vi "p1.vi"() -> ()   [LabVIEW 2023, in "d19.lvlib"]
uses:
  d19.lvlib
  Users/Standard/OneDrive - Argenta/Desktop/SubPanel Actors/GUI/GUI/Rule Type.ctl
  <vilib>/regexp/Match Regular Expression.xnode
  AOC/AOC.lvlib
panel:
  in  "Example":string="px{a<2006:qkq,m>2090:A,rfg}\npv{a>1716:R,A}\nlnx{m>1548:A,A}\nrfg{s<537:gd,x>2440:R,A}\nqs{s>3448:A,lnx}\nqkq{x<1416:A,crn}\ncrn{x>2662:A,R}\nin{s<1351:px,qqz}\nqqz{s>2770:qs,m<1801:hdj,R}\ngd{a>3333:R,R}\nhdj{m>838:A,pv}\n\n{x=787,m=2655,a=1222,s=2876}\n{x=1679,m=44,a=2067,s=496}\n{x=2036,m=264,a=79,s=2244}\n{x=2461,m=1339,a=466,s=291}\n{x=2127,m=1623,a=2188,s=1013}"
  in  "Example":bool=TRUE
  out "Answer":i64=978
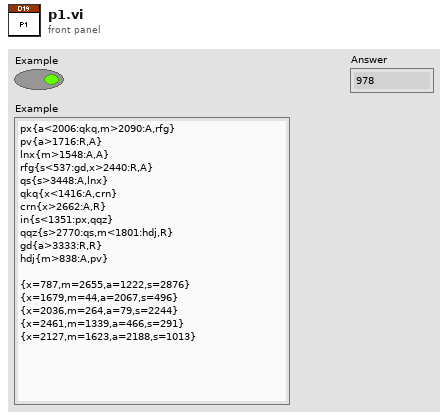
[diagram p1: front panel]
types:
  T1 = cluster{"Rule Type":string, "Index":i32, "Label":string}[]
  T2 = typedef "d19.lvlib/Rule Type.ctl" = enum16{"<", ">", "R", "A", "goto"}
  T3 = map{string, cluster{"Type":T2, "Route":string, "Rating":u8, "Value":i32}[]}
  T4 = cluster{"Type":T2, "whole match":string, "default value 1":u8, i32}
  T5 = cluster{"Type":T2, "Route":string, "Rating":u8, "Value":i32}[]
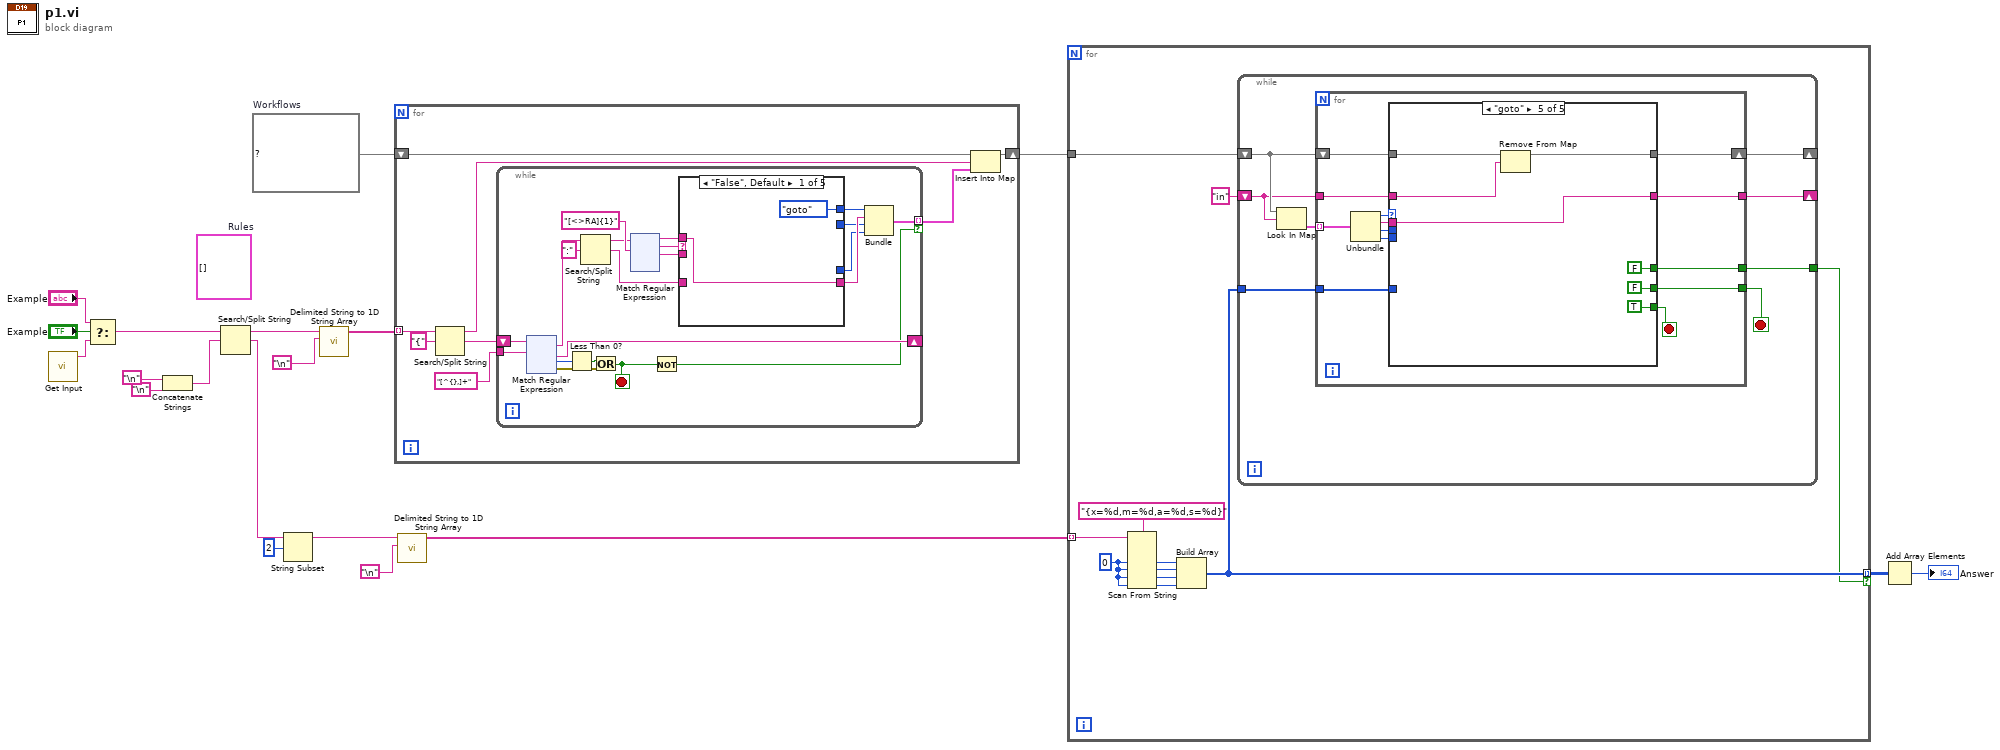
[diagram p0: block diagram]
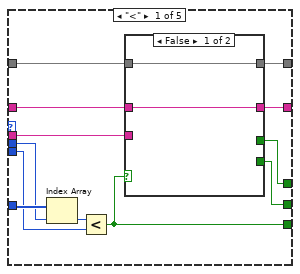
[diagram p2: hidden frame]
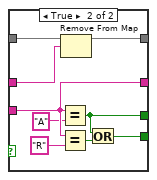
[diagram p3: hidden frame]
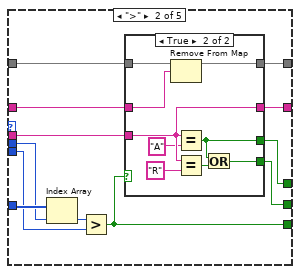
[diagram p4: hidden frame]
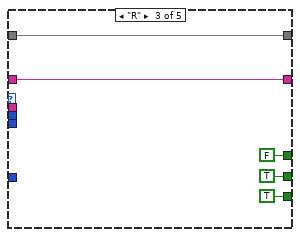
[diagram p6: hidden frame]
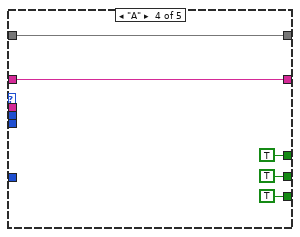
[diagram p7: hidden frame]
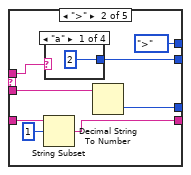
[diagram p8: hidden frame]
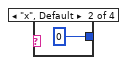
[diagram p9: hidden frame]
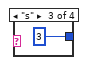
[diagram p10: hidden frame]
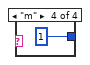
[diagram p11: hidden frame]
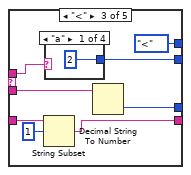
[diagram p12: hidden frame]
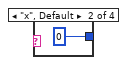
[diagram p13: hidden frame]
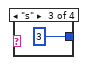
[diagram p14: hidden frame]
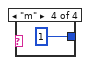
[diagram p15: hidden frame]
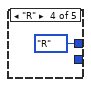
[diagram p16: hidden frame]
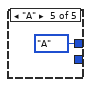
[diagram p17: hidden frame]
diagram:
  (unwired) T1 []  # Rules
  w9 = T3 {}  # Workflows
  n1 = call "Get Input.vi"() -> ("Input"=w19:string)  [unwired: 11 in]
  n2 = Select(t="Example", s="Example", f=w19) -> (s? t:f=w16:string)
  n3 = Concatenate Strings("\n", "\n") -> (w13:string)
  n4 = Search/Split String(string=w16, search string/char (-)=w13) -> (substring before match=w12:string, match + rest of string=w11:string)  [unwired: 1 in, 1 out]
  n5 = String Subset(string=w11, offset (0)=2) -> (substring=w2:string)  [unwired: 1 in]
  n6 = call <vilib>:"Delimited String to 1D String Array.vi"("delimiter"="\n", "delimited string"=w12) -> ("string array"=w10:string[])  [unwired: 9 in]
  n7 = for {
    tunnel: w10 -> [w25] mode=indexing
    shift-right: [w26] -> w5
    shift-left: w9 -> [w27]
    n8 = Search/Split String(string=w25, search string/char (-)="{") -> (substring before match=w23:string, match + rest of string=w22:string)  [unwired: 1 in, 1 out]
    n9 = while {
      shift-right: [w47] -> _
      shift-left: w22 -> [w48]
      tunnel: [w32] -> w20 mode=indexing if=w41
      tunnel: "[^{},]+" -> [w46]
      stop <- w42 stop-if-true
      n10 = xnode "Match Regular Expression"("input string"=w48, "regular expression"=w46) -> ("whole match"=w30:string, "after match"=w47:string, "offset past match"=w45:i32, "error out"=w43:errorcluster)  [unwired: 4 in, 1 out]
      n11 = Less Than 0?(x=w45) -> (x < 0?=w44:bool)
      n12 = Search/Split String(string=w30, search string/char (-)=":") -> (substring before match=w29:string, match + rest of string=w28:string)  [unwired: 1 in, 1 out]
      n13 = Or(x=w44, y=w43) -> (x .or. y?=w42:bool)
      n14 = xnode "Match Regular Expression"("input string"=w29, "regular expression"="[<>RA]{1}") -> ("before match"=w38:string, "whole match"=w39:string, "after match"=w37:string)  [unwired: 4 in, 2 out]
      n15 = Not(x=w42) -> (.not. x?=w41:bool)
      n16 = case shown="\"False\", Default" w39 {
        tunnel: [Rule_Type."goto" ("Type") Rule_Type.">" ("Type") Rule_Type."<" ("Type") Rule_Type."R" ("Type") Rule_Type."A" ("Type")] -> w36
        tunnel: w38 -> [w50 w56 w68 _ _]
        tunnel: w37 -> [_ w54 w66 _ _]
        tunnel: [_ w55 w67 _ _] -> w34
        tunnel: [_ w57 w69 _ _] -> w33
        tunnel: [w50 w52 w64 _ _] -> w35
        tunnel: w28 -> [_ w53 w65 _ _]
        frame "False", Default {
        }
        frame ">" {
          n17 = String Subset(string=w53, offset (0)=1) -> (substring=w52:string)  [unwired: 1 in]
          n18 = case shown="\"a\"" w56 {
            tunnel: [u8 2 ("default value 1") u8 0 ("default value 1") u8 3 ("default value 1") u8 1 ("default value 1")] -> w55
            frame "a" {
            }
            frame "x", Default {
            }
            frame "s" {
            }
            frame "m" {
            }
          }
          n19 = Decimal String To Number(string=w54) -> (number=w57:i32)  [unwired: 2 in, 1 out]
        }
        frame "<" {
          n20 = String Subset(string=w65, offset (0)=1) -> (substring=w64:string)  [unwired: 1 in]
          n21 = case shown="\"a\"" w68 {
            tunnel: [u8 2 ("default value 1") u8 0 ("default value 1") u8 3 ("default value 1") u8 1 ("default value 1")] -> w67
            frame "a" {
            }
            frame "x", Default {
            }
            frame "s" {
            }
            frame "m" {
            }
          }
          n22 = Decimal String To Number(string=w66) -> (number=w69:i32)  [unwired: 2 in, 1 out]
        }
        frame "R" {
        }
        frame "A" {
        }
      }
      n23 = Bundle("Type"=w36, "whole match"=w35, "default value 1"=w34, w33) -> (w32:T4)  [unwired: 1 in]
    }
    n24 = Insert Into Map(map in=w27, key=w23, value=w20) -> (map out=w26:T3)  [unwired: 2 out]
  }
  n25 = call <vilib>:"Delimited String to 1D String Array.vi"("delimiter"="\n", "delimited string"=w2) -> ("string array"=w8:string[])  [unwired: 9 in]
  n26 = for {
    tunnel: w8 -> [w321] mode=indexing
    tunnel: w5 -> [w319]
    tunnel: [w312] -> w4 mode=indexing if=w311
    w313 = i64 0 ("default value 1")
    n27 = Scan From String(format string="{x=%d,m=%d,a=%d,s=%d}", input string=w321, default 1=w313, default 2=w313, default 3=w313, default 4=w313) -> (output 1=w317:i64, output 2=w316:i64, output 3=w315:i64, output 4=w314:i64)  [unwired: 2 in, 3 out]
    n28 = Build Array(w317, w316, w315, w314) -> (w312:i64[])
    n29 = while {
      shift-right: [w327] -> _
      shift-left: "in" -> [w326]
      shift-right: [w322] -> _
      shift-left: w319 -> [w328]
      tunnel: w312 -> [w325]
      tunnel: [w323] -> w311
      stop <- w324 stop-if-true
      n30 = Look In Map(map=w328, key=w326) -> (value=w329:T5)  [unwired: 1 in, 1 out]
      n31 = for {
        tunnel: w329 -> [w342] mode=indexing
        tunnel: w325 -> [w333]
        shift-right: [w330] -> w322
        shift-left: w328 -> [w337]
        tunnel: [w336] -> w327
        tunnel: w326 -> [w334]
        tunnel: [w332] -> w324
        tunnel: [w331] -> w323
        stop <- w335 stop-if-true
        n32 = Unbundle(w342) -> ("Type"=w341:T2, "Route"=w340:string, "Rating"=w339:u8, "Value"=w338:i32)
        n33 = case shown="\"goto\"" w341 {
          tunnel: w333 -> [w354 w377 _ _ _]
          tunnel: w340 -> [w350 w373 _ _ w402]
          tunnel: w339 -> [w353 w376 _ _ _]
          tunnel: w338 -> [w351 w374 _ _ _]
          tunnel: w337 -> [w344 w367 w389 w394 w401]
          tunnel: [w349 w372 w390 w395 w402] -> w336
          tunnel: [w348 w371 TRUE TRUE TRUE] -> w335
          tunnel: w334 -> [w347 w370 w390 w395 w399]
          tunnel: [w345 w368 TRUE TRUE FALSE] -> w332
          tunnel: [w346 w369 FALSE TRUE FALSE] -> w331
          tunnel: [w343 w366 w389 w394 w400] -> w330
          frame "<" {
            n34 = Index Array(array=w354, index=w353) -> (element=w352:i64)
            n35 = Less?(x=w352, y=w351) -> (x < y?=w348:bool)
            n36 = case shown="False" w348 {
              tunnel: w350 -> [_ w365]
              tunnel: [w356 w365] -> w349
              tunnel: w347 -> [w356 w357]
              tunnel: [_ w363] -> w346
              tunnel: [_ w361] -> w345
              tunnel: w344 -> [w355 w359]
              tunnel: [w355 w358] -> w343
              frame False {
              }
              frame True {
                n37 = Equal?(x=w365, y="A") -> (x = y?=w363:bool)
                n38 = Equal?(x=w365, y="R") -> (x = y?=w362:bool)
                n39 = Remove From Map(10:w357, 11:w359) -> (3:w358:T3)  [unwired: 2 out]
                n40 = Or(x=w363, y=w362) -> (x .or. y?=w361:bool)
              }
            }
          }
          frame ">" {
            n41 = Index Array(array=w377, index=w376) -> (element=w375:i64)
            n42 = Greater?(x=w375, y=w374) -> (0:w371:bool)
            n43 = case shown="True" w371 {
              tunnel: w373 -> [_ w388]
              tunnel: [w379 w388] -> w372
              tunnel: w370 -> [w379 w380]
              tunnel: [_ w386] -> w369
              tunnel: [_ w384] -> w368
              tunnel: w367 -> [w378 w382]
              tunnel: [w378 w381] -> w366
              frame False {
              }
              frame True {
                n44 = Remove From Map(10:w380, 11:w382) -> (3:w381:T3)  [unwired: 2 out]
                n45 = Equal?(x=w388, y="A") -> (x = y?=w386:bool)
                n46 = Equal?(x=w388, y="R") -> (x = y?=w385:bool)
                n47 = Or(x=w386, y=w385) -> (x .or. y?=w384:bool)
              }
            }
          }
          frame "R" {
          }
          frame "A" {
          }
          frame "goto" {
            n48 = Remove From Map(10:w399, 11:w401) -> (3:w400:T3)  [unwired: 2 out]
          }
        }
      }
    }
  }
  n49 = Add Array Elements(numeric array=w4) -> (sum=→"Answer":i64)
